vi "add tag.vi"(7 "owner ID":string, 8 "error in":errorcluster, 10 "tag descriptor":refnum<class "tag descriptor.lvclass">, 11 "engine configuration in":refnum<class "engine configuration.lvclass">) -> (0 "error out":errorcluster, 3 "engine configuration out":refnum<class "engine configuration.lvclass">)   [LabVIEW 2013, in "engine configuration.lvclass"]
doc: "This function adds a tag to the engine configuration. The owner ID is an optional field used to specify who has permission to modify the tag. An empty string is used to specify that anyone has permission to make modifications."
uses:
  engine configuration.lvclass
  <vilib>/NI/Tag Bus/tag/tag descriptor.lvclass
  <vilib>/NI/Tag Bus/tag/tag descriptor.lvclass/tag descriptor.ctl
  module channel pairings.ctl
  engine configuration.lvclass/engine configuration.ctl
  <vilib>/NI/Configuration Framework/NISE_CEF_TreeControl.lvlib
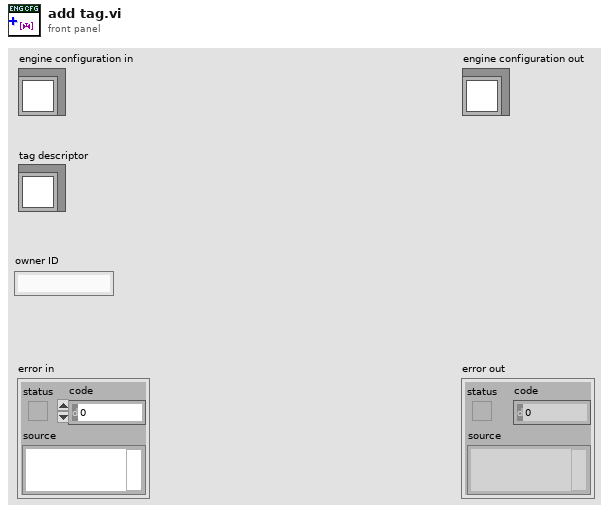
[diagram p1: front panel]
types:
  T1 = typedef "engine configuration.lvclass/module channel pairings.ctl" = cluster{"modules":string[], "channels":string[]}
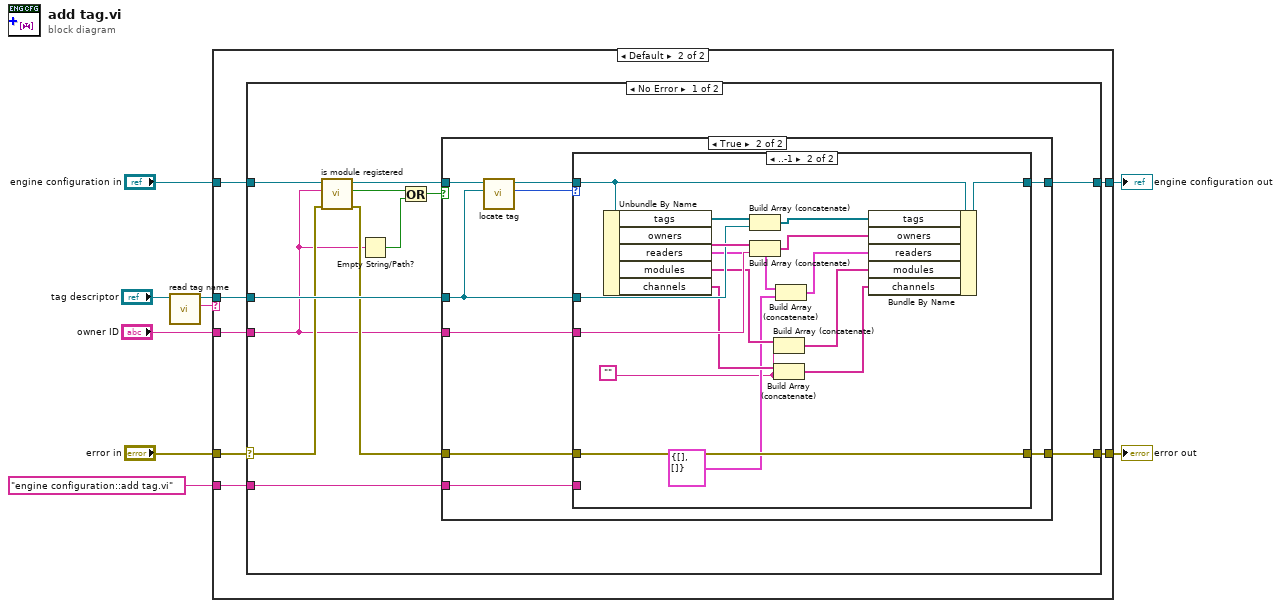
[diagram p0: block diagram]
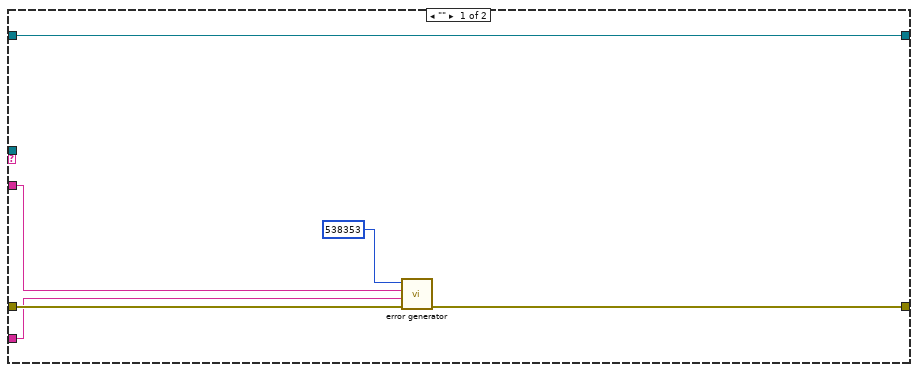
[diagram p2: hidden frame]
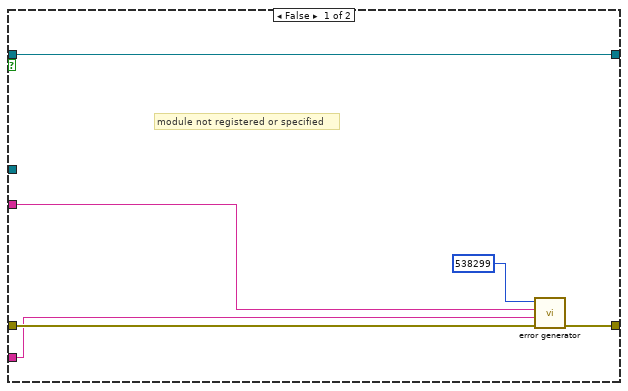
[diagram p3: hidden frame]
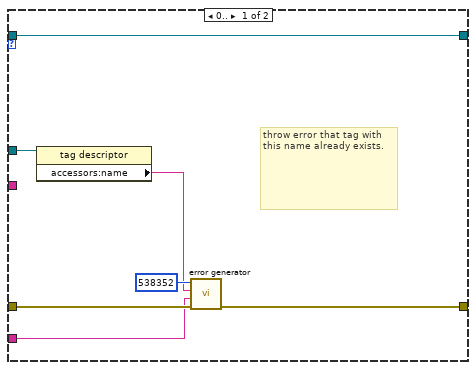
[diagram p4: hidden frame]
diagram:
  n1 = call <vilib>:"read tag name.vi"("system tag in"="tag descriptor") -> ("name"=w2:string, "system tag out"=w3:refnum<class "tag descriptor.lvclass">)  [unwired: 8 in, 1 out]
  n2 = case shown="Default" w2 {
    tunnel: "error in" -> [w14 w22]
    tunnel: [w13 w21] -> w8
    tunnel: "engine configuration in" -> [w15 w20]
    tunnel: [w15 w19] -> w6
    tunnel: "owner ID" -> [w11 w18]
    tunnel: w3 -> [_ w17]
    tunnel: "engine configuration::add tag.vi" ("source") -> [w10 w16]
    frame "" {
      n3 = call <vilib>:"error generator.vi"("error in"=w14, "source"=w10, "append error message"=w11, "error code (0)"=538353) -> ("error out"=w13:errorcluster)  [unwired: 5 in]
    }
    frame Default {
      n4 = case shown="No Error" w22 {
        selector: w22 -> [w29 w75]
        tunnel: [w33 w75] -> w21
        tunnel: [w34 w74] -> w19
        tunnel: w20 -> [w31 w74]
        tunnel: w17 -> [w32 _]
        tunnel: w18 -> [w24 _]
        tunnel: w16 -> [w23 _]
        frame No Error {
          n5 = call-dynamic "is module registered.vi"("error in"=w29, "module ID"=w24, "engine configuration in"=w31) -> ("error out"=w28:errorcluster, "registered?"=w27:bool, "engine configuration out"=w30:refnum<class "engine configuration.lvclass">)  [unwired: 6 in]
          n6 = Empty String/Path?(string/path=w24) -> (empty?=w25:bool)
          n7 = Or(x=w27, y=w25) -> (x .or. y?=w26:bool)
          n8 = case shown="True" w26 {
            tunnel: [w40 w47] -> w34
            tunnel: [w38 w46] -> w33
            tunnel: w32 -> [_ w45]
            tunnel: w30 -> [w40 w44]
            tunnel: w28 -> [w39 w43]
            tunnel: w24 -> [w36 w42]
            tunnel: w23 -> [w35 w41]
            frame False {
              # "module not registered or specified"
              n9 = call <vilib>:"error generator.vi"("error in"=w39, "source"=w35, "append error message"=w36, "error code (0)"=538299) -> ("error out"=w38:errorcluster)  [unwired: 5 in]
            }
            frame True {
              n10 = call "locate tag.vi"("tag descriptor"=w45, "engine configuration in"=w44) -> ("index"=w49:i32, "engine configuration out"=w48:refnum<class "engine configuration.lvclass">)  [unwired: 8 in]
              n11 = case shown="..-1" w49 {
                tunnel: w48 -> [w56 w71]
                tunnel: [w56 w69] -> w47
                tunnel: w43 -> [w54 w73]
                tunnel: [w53 w73] -> w46
                tunnel: w45 -> [w52 w65]
                tunnel: w42 -> [_ w66]
                tunnel: w41 -> [w50 _]
                frame 0.. {
                  # "throw error that tag with this name already exists."
                  n12 = property class="tag descriptor"(reference=w52) -> ("accessors:name"=w51:string)  [unwired: 1 in, 2 out]
                  n13 = call <vilib>:"error generator.vi"("error in"=w54, "source"=w50, "append error message"=w51, "error code (0)"=538352) -> ("error out"=w53:errorcluster)  [unwired: 5 in]
                }
                frame ..-1 {
                  w57 = ""
                  n14 = Unbundle By Name(w71) -> ("tags"=w72:refnum<class "tag descriptor.lvclass">[], "owners"=w68:string[], "readers"=w60:T1[], "modules"=w61:string[], "channels"=w62:string[])
                  n15 = Build Array (concatenate)(w72, w65) -> (w70:refnum<class "tag descriptor.lvclass">[])
                  n16 = Build Array (concatenate)(w68, w66) -> (w67:string[])
                  n17 = Build Array (concatenate)(w61, w57) -> (w64:string[])
                  n18 = Build Array (concatenate)(w62, w57) -> (w63:string[])
                  n19 = Build Array (concatenate)(w60, T1 {"modules"=[], "channels"=[]} ("cluster of array of strings")) -> (w59:T1[])
                  n20 = Bundle By Name(cluster=w71, "tags"=w70, "owners"=w67, "readers"=w59, "modules"=w64, "channels"=w63) -> (w69:refnum<class "engine configuration.lvclass">)
                }
              }
            }
          }
        }
        frame Error {
        }
      }
    }
  }
  "error out" <- w8
  "engine configuration out" <- w6
